vi "UpdateSample.vi"(8 "error in (no error)":errorcluster, 11 "DB in":refnum<class "DB.lvclass">) -> (0 "error out":errorcluster, 3 "DB out":refnum<class "DB.lvclass">)   [LabVIEW 2020, in "DB.lvclass"]
uses:
  DB.lvclass
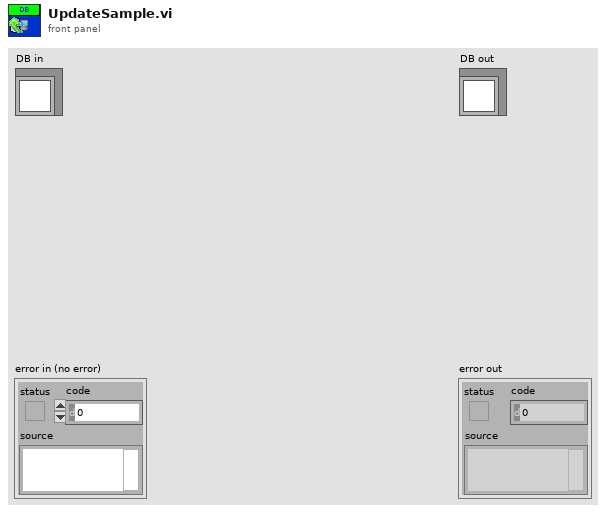
[diagram p1: front panel]
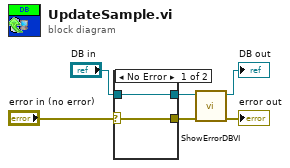
[diagram p0: block diagram]
diagram:
  n1 = case shown="No Error" "error in (no error)" {
    selector: "error in (no error)" -> [w7 w10]
    tunnel: [w7 w10] -> w4
    tunnel: [w8 w9] -> w2
    tunnel: "DB in" -> [w8 w9]
    frame No Error {
    }
    frame Error {
    }
  }
  n2 = call "ShowErrorDBVI.vi"("error in (no error)"=w4, "DB in"=w2) -> ("error out"=→"error out":errorcluster, "DB out"=→"DB out":refnum<class "DB.lvclass">)  [unwired: 8 in]
